vi "Read State.vi"(0 "VISA resource name":refnum<visa-resource-name>, 11 "error in (no error)":errorcluster) -> (4 "VISA resource name out":refnum<visa-resource-name>, 6 "State":string, 15 "error out":errorcluster)   [LabVIEW 2014, in "Associated Power Technologies 8500 Series.lvlib"]
doc: "Gets the instrument state."
uses:
  <instrlib>/Associated Power Technologies 8500 Series/Associated Power Technologies 8500 Series.lvlib
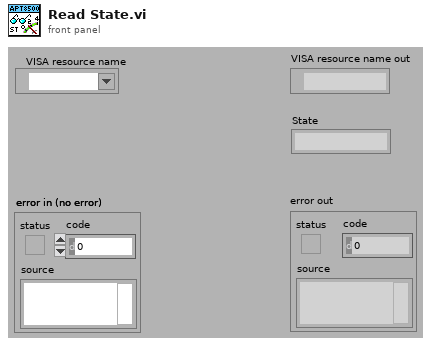
[diagram p1: front panel]
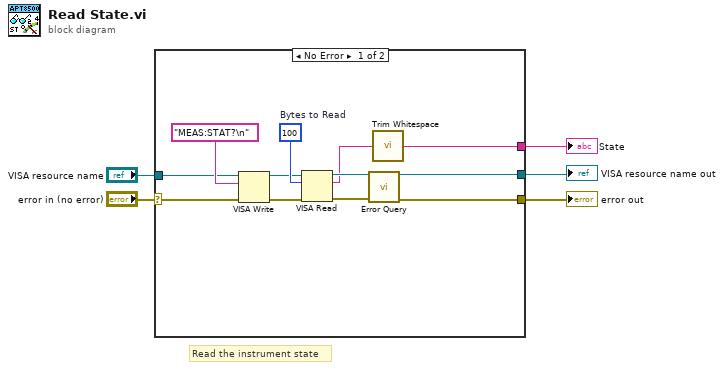
[diagram p0: block diagram]
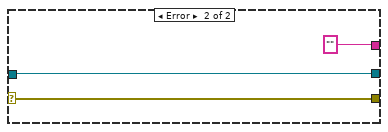
[diagram p2: hidden frame]
diagram:
  # "Read the instrument state"
  n1 = case shown="No Error" "error in (no error)" {
    selector: "error in (no error)" -> [w13 w20]
    tunnel: [w8 w20] -> w4
    tunnel: [w11 w19] -> w2
    tunnel: "VISA resource name" -> [w12 w19]
    tunnel: [w6 ""] -> w1
    frame No Error {
      w17 = u32 100  # Bytes to Read
      n2 = VISA Write(VISA resource name=w12, write buffer="MEAS:STAT?\n", error in (no error)=w13) -> (VISA resource name out=w15:refnum<visa-resource-name>, error out=w16:errorcluster)  [unwired: 1 out]
      n3 = VISA Read(VISA resource name=w15, byte count=w17, error in (no error)=w16) -> (VISA resource name out=w10:refnum<visa-resource-name>, read buffer=w7:string, error out=w9:errorcluster)  [unwired: 1 out]
      n4 = call <instrlib>:"Error Query.vi"("VISA resource name"=w10, "error in (no error)"=w9) -> ("VISA resource name out"=w11:refnum<visa-resource-name>, "error out"=w8:errorcluster)  [unwired: 10 in, 2 out]
      n5 = call <vilib>:"Trim Whitespace.vi"("string"=w7) -> ("trimmed string"=w6:string)  [unwired: 1 in]
    }
    frame Error {
    }
  }
  "error out" <- w4
  "VISA resource name out" <- w2
  "State" <- w1
